vi "PPS Init.vi"(8 "error in (no error)":errorcluster, 10 "VISA resource name":refnum<visa-resource-name>, 11 "IT-M3904D in":refnum<class "IT-M3904D.lvclass">) -> (0 "error out":errorcluster, 3 "IT-M3904D out":refnum<class "IT-M3904D.lvclass">)   [LabVIEW 2023, in "HardwareAbstractionLayer_LVOOP.lvlib" / "IT-M3904D.lvclass"]
uses:
  IT-M3904D.lvclass
  PowerSupply.lvclass
  <instrlib>/IT-M3900D/IT-M3900D.lvlib
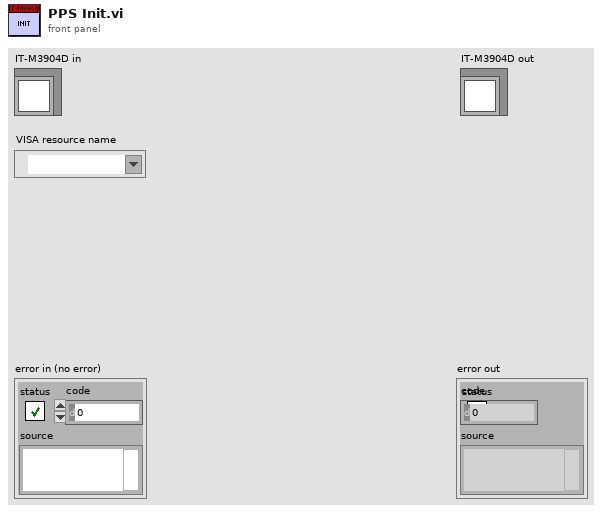
[diagram p1: front panel]
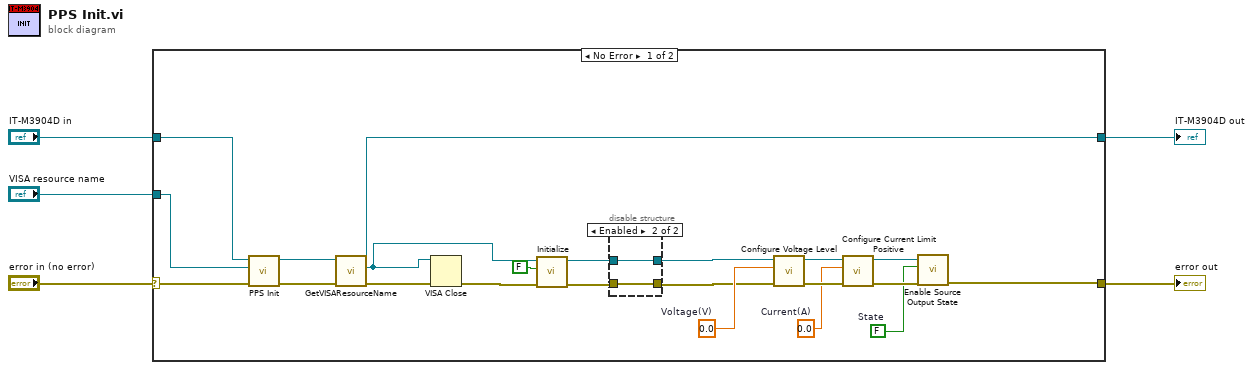
[diagram p0: block diagram]
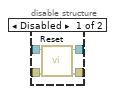
[diagram p2: hidden frame]
diagram:
  n1 = case shown="No Error" "error in (no error)" {
    selector: "error in (no error)" -> [w27 w35]
    tunnel: [w13 w35] -> w4
    tunnel: "VISA resource name" -> [w16 _]
    tunnel: "IT-M3904D in" -> [w26 w34]
    tunnel: [w14 w34] -> w1
    frame No Error {
      w17 = FALSE  # State
      w18 = 0.0  # Current(A)
      w19 = 0.0  # Voltage(V)
      n2 = call-parent "PPS Init.vi"("error in (no error)"=w27, "VISA resource name"=w16, "PowerSupply in"=w26) -> ("error out"=w25:errorcluster, "PowerSupply out"=w24:refnum<class "IT-M3904D.lvclass">)  [unwired: 7 in]
      n3 = call "GetVISAResourceName.vi"("error in (no error)"=w25, "object in"=w24) -> ("error out"=w7:errorcluster, "VISA resource name"=w8:refnum<visa-resource-name>, "object out"=w14:refnum<class "IT-M3904D.lvclass">)  [unwired: 7 in]
      n4 = VISA Close(VISA resource name=w8, error in (no error)=w7) -> (error out=w6:errorcluster)
      n5 = call <instrlib>:"Initialize.vi"("error in"=w6, "ID Query"=FALSE, "VISA resource name"=w8) -> ("error out"=w10:errorcluster, "VISA resource name out"=w12:refnum<visa-resource-name>)  [unwired: 7 in]
      n6 = disable-structure shown="Enabled" {
        disable-tunnel: w12 -> [w31 w33]
        disable-tunnel: [w30 w33] -> w11
        disable-tunnel: w10 -> [w29 w32]
        disable-tunnel: [w28 w32] -> w9
        frame Disabled {
          n7 = call <instrlib>:"Reset.vi"("error in"=w29, "VISA resource name"=w31) -> ("error out"=w28:errorcluster, "VISA resource name out"=w30:refnum<visa-resource-name>)  [unwired: 8 in]
        }
        frame Enabled {
        }
      }
      n8 = call <instrlib>:"Configure Voltage Level.vi"("error in"=w9, "Voltage(V)"=w19, "VISA resource name"=w11) -> ("error out"=w22:errorcluster, "VISA resource name out"=w23:refnum<visa-resource-name>)  [unwired: 7 in]
      n9 = call <instrlib>:"Configure Current Limit Positive.vi"("error in"=w22, "Value(A)"=w18, "VISA resource name"=w23) -> ("error out"=w20:errorcluster, "VISA resource name out"=w21:refnum<visa-resource-name>)  [unwired: 7 in]
      n10 = call <instrlib>:"Enable Source Output State.vi"("error in"=w20, "State"=w17, "VISA resource name"=w21) -> ("error out"=w13:errorcluster)  [unwired: 7 in, 1 out]
    }
    frame Error {
    }
  }
  "error out" <- w4
  "IT-M3904D out" <- w1
